vi "New Create Cal File Array (RIO).vi"() -> (0 "Cal Target Array":string[](array[string]), 3 "Cal Log OUT":string[][](array[string]))   [LabVIEW 2019]
uses:
  Type Defs/Units Type Def (DAQ Rack).ctl
  Type Defs/New Channel Type Def (RIO).ctl
panel:
  in  "Channel to Cal":T1
  in  "Cal Unit":T2
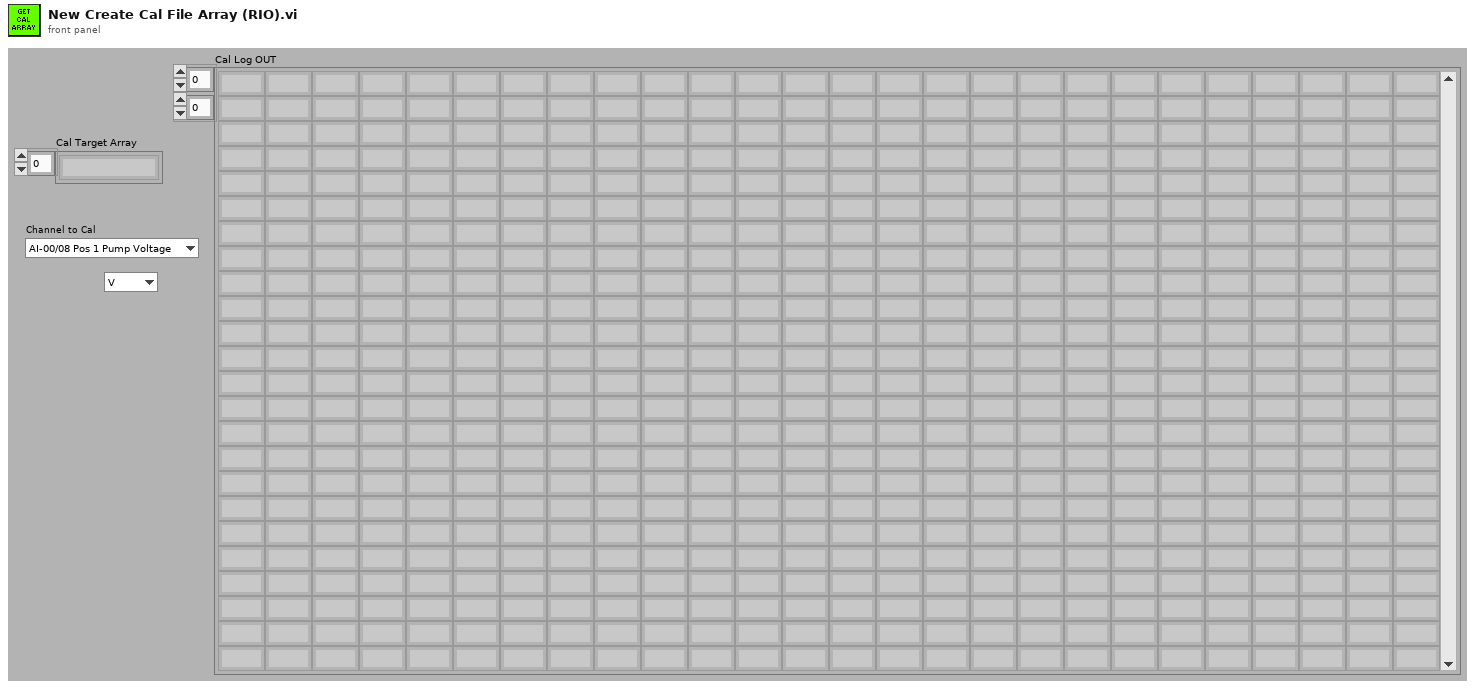
[diagram p1: front panel]
types:
  T1 = typedef "New Channel Type Def (RIO).ctl" = enum16{"AI-00/08 Pos 1 Pump Voltage", "AI-01/09 Pos 2 Pump Voltage", "AI-02/10 Pos 3 Pump Voltage", "AI-03/11 Pos 4 Pump Voltage", "AI-04/12 Pos 5 Pump Voltage", "AI-05/13 Pos 6 Pump Voltage", "AI-06 Spare", "AI-14 Spare", "AI-07 Spare", "AI-15 Power Supply Voltage", "AI-16 Pos 1 Pump Current", "AI-17 Pos 2 Pump Current", "AI-18 Pos 3 Pump Current", "AI-19 Pos 4 Pump Current", "AI-20 Pos 5 Pump Current", "AI-21 Pos 6 Pump Current", "AI-16 Pos 1 Pump Speed", "AI-17 Pos 2 Pump Speed", "AI-18 Pos 3 Pump Speed", "AI-19 Pos 4 Pump Speed", "AI-20 Pos 5 Pump Speed", "AI-21 Pos 6 Pump Speed", "AI-22 Pos 1 Controller Current", "AI-23 Pos 2 Controller Current", "AI-24 Pos 3 Controller Current", "AI-25 Pos 4 Controller Current", "AI-26 Pos 5 Controller Current", "AI-27 Pos 6 Controller Current", "AI-28 Tank 1 Temperature", "AI-29 Tank 2 Temperature", "AI-30 Pos 1 Pump Pressure", "AI-31 Pos 2 Pump Pressure", "AI-32 Pos 3 Pump Pressure", "AI-33 Pos 4 Pump Pressure", "AI-34 Pos 5 Pump Pressure", "AI-35 Pos 6 Pump Pressure", "AI-36 Pos 1 Pump Flow", "AI-37 Pos 2 Pump Flow", "AI-38 Pos 3 Pump Flow", "AI-39 Pos 4 Pump Flow", "AI-40 Pos 5 Pump Flow", "AI-41 Pos 6 Pump Flow", "AI-42 Spare", "AI-43 Spare", "AI-44 Spare", "AI-45 Spare", "AI-46 Spare", "AI-47 Spare", "AI-00/08 Pos 1 Controller Voltage", "AI-01/09 Pos 2 Controller Voltage", "AI-02/10 Pos 3 Controller Voltage", "AI-03/11 Pos 4 Controller Voltage", "AI-04/12 Pos 5 Controller Voltage", "AI-05/13 Pos 6 Controller Voltage"}
  T2 = typedef "Units Type Def (DAQ Rack).ctl" = enum16{"V", "mA", "A", "Hz", "deg C"}
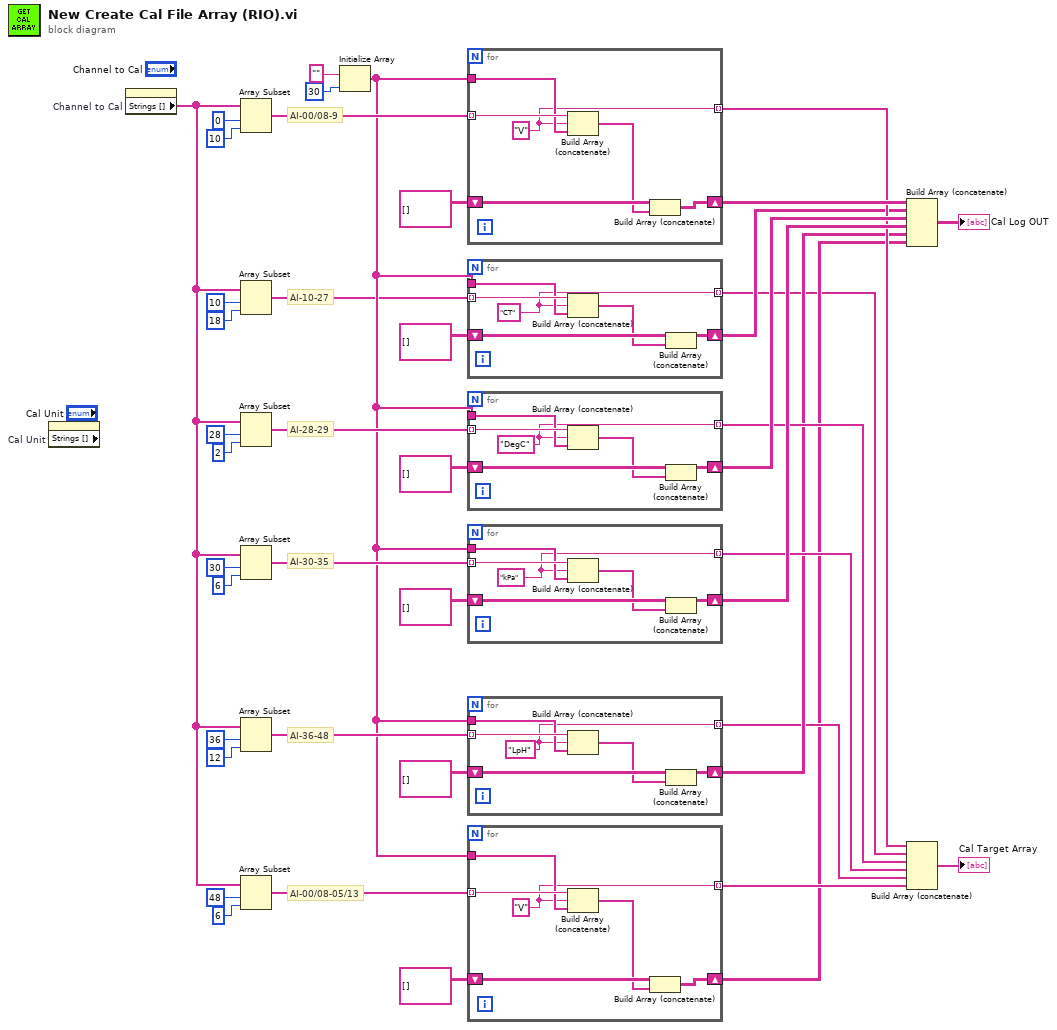
[diagram p0: block diagram]
diagram:
  # "AI-10-27"
  # "AI-00/08-05/13"
  # "AI-36-48"
  # "AI-30-35"
  # "AI-28-29"
  # "AI-00/08-9"
  n1 = property on="Cal Unit" class="Enum (strict)" props=["Strings []"]() -> ()  [unwired: 2 in, 3 out]
  n2 = property on="Channel to Cal" class="Enum (strict)"() -> ("Strings []"=w3:string[])  [unwired: 2 in, 2 out]
  n3 = Array Subset(array=w3, index=0, length=10) -> (w38:string[])
  n4 = Array Subset(array=w3, index=10, length=18) -> (w4:string[])
  n5 = Array Subset(array=w3, index=28, length=2) -> (w33:string[])
  n6 = Array Subset(array=w3, index=30, length=6) -> (w22:string[])
  n7 = Array Subset(array=w3, index=36, length=12) -> (w23:string[])
  n8 = Array Subset(array=w3, index=48, length=6) -> (w11:string[])
  n9 = Initialize Array("", 30 ("dimension size")) -> (w7:string[])
  n10 = for {
    tunnel: w38 -> [w48] mode=indexing
    tunnel: w7 -> [w47]
    shift-right: [w45] -> w32
    shift-left: string[][] [] ("Cal Log OUT") -> [w46]
    tunnel: [w43] -> w18 mode=indexing
    w43 = "V"
    n11 = Build Array (concatenate)(w48, w43, w47) -> (w44:string[])
    n12 = Build Array (concatenate)(w46, w44) -> (w45:string[][])
  }
  n13 = for {
    tunnel: w4 -> [w52] mode=indexing
    tunnel: w7 -> [w50]
    shift-right: [w53] -> w2
    shift-left: string[][] [] ("Cal Log OUT") -> [w54]
    tunnel: [w49] -> w1 mode=indexing
    w49 = "CT"
    n14 = Build Array (concatenate)(w52, w49, w50) -> (w51:string[])
    n15 = Build Array (concatenate)(w54, w51) -> (w53:string[][])
  }
  n16 = for {
    tunnel: w33 -> [w58] mode=indexing
    tunnel: w7 -> [w56]
    shift-right: [w59] -> w30
    shift-left: string[][] [] ("Cal Log OUT") -> [w60]
    tunnel: [w55] -> w17 mode=indexing
    w55 = "DegC"
    n17 = Build Array (concatenate)(w58, w55, w56) -> (w57:string[])
    n18 = Build Array (concatenate)(w60, w57) -> (w59:string[][])
  }
  n19 = for {
    tunnel: w22 -> [w64] mode=indexing
    tunnel: w7 -> [w62]
    shift-right: [w65] -> w21
    shift-left: string[][] [] ("Cal Log OUT") -> [w66]
    tunnel: [w61] -> w19 mode=indexing
    w61 = "kPa"
    n20 = Build Array (concatenate)(w64, w61, w62) -> (w63:string[])
    n21 = Build Array (concatenate)(w66, w63) -> (w65:string[][])
  }
  n22 = for {
    tunnel: w23 -> [w70] mode=indexing
    tunnel: w7 -> [w68]
    shift-right: [w71] -> w16
    shift-left: string[][] [] ("Cal Log OUT") -> [w72]
    tunnel: [w67] -> w15 mode=indexing
    w67 = "LpH"
    n23 = Build Array (concatenate)(w70, w67, w68) -> (w69:string[])
    n24 = Build Array (concatenate)(w72, w69) -> (w71:string[][])
  }
  n25 = for {
    tunnel: w11 -> [w78] mode=indexing
    tunnel: w7 -> [w77]
    shift-right: [w75] -> w9
    shift-left: string[][] [] ("Cal Log OUT") -> [w76]
    tunnel: [w73] -> w10 mode=indexing
    w73 = "V"
    n26 = Build Array (concatenate)(w78, w73, w77) -> (w74:string[])
    n27 = Build Array (concatenate)(w76, w74) -> (w75:string[][])
  }
  n28 = Build Array (concatenate)(w32, w2, w30, w21, w16, w9) -> (→"Cal Log OUT":string[][])
  n29 = Build Array (concatenate)(w18, w1, w17, w19, w15, w10) -> (→"Cal Target Array":string[])
